vi "Write Objects.vi"(8 "error in (no error)":errorcluster, 10 "objects":cluster{"object ID":u8, "value":string}[](array[cluster]) {"object ID" format="%x"}, 11 "standard data model in":refnum<class "Standard Data Model.lvclass">) -> (0 "error out":errorcluster, 3 "standard data model out":refnum<class "Standard Data Model.lvclass">)   [LabVIEW 2017, in "SubVIs.lvlib" / "Standard Data Model.lvclass"]
doc: "Writes objects to the device model."
uses:
  <vilib>/Modbus/subvis/Data and Functions/Standard Data Model/Standard Data Model.lvclass
  <vilib>/Modbus/subvis/Data and Functions/Standard Data Model/Standard Data Model.lvclass/Standard Data Model.ctl
  <vilib>/Modbus/subvis/Data and Functions/Device Data Model/Device Data Model.lvclass
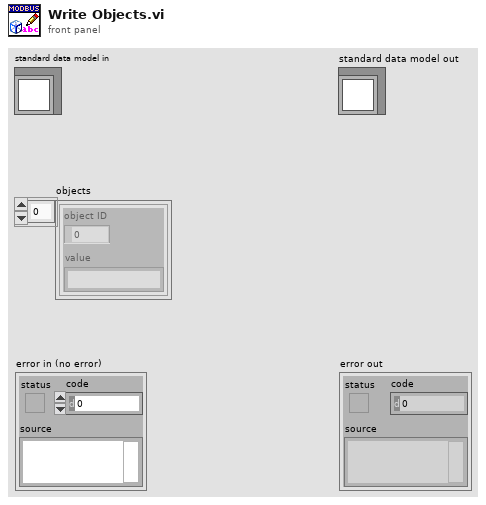
[diagram p1: front panel]
types:
  T1 = typedef "SubVIs.lvlib/Device Data Model.lvclass/Identification Parameters.ctl" = cluster{"object ID":u8, "value":string}
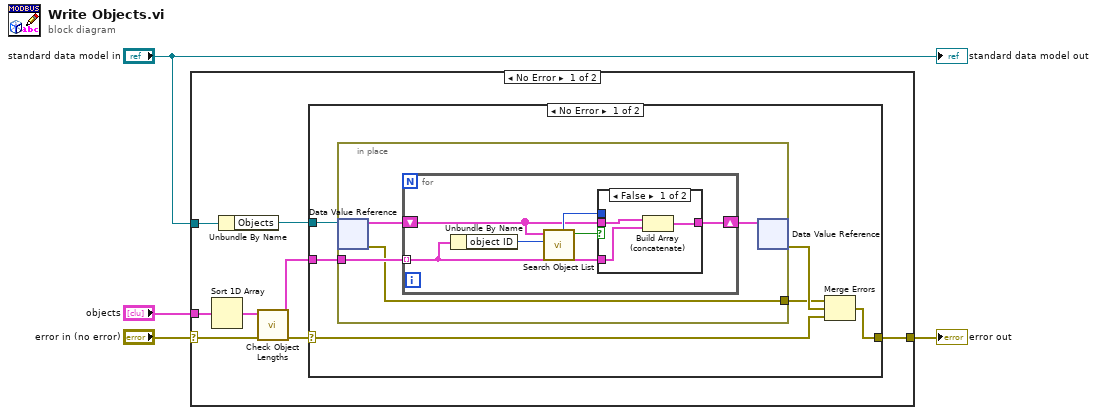
[diagram p0: block diagram]
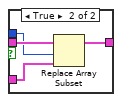
[diagram p2: hidden frame]
diagram:
  n1 = case shown="No Error" "error in (no error)" {
    selector: "error in (no error)" -> [w5 w37]
    tunnel: "objects" -> [w12 _]
    tunnel: "standard data model in" -> [w10 _]
    tunnel: [w7 w37] -> w2
    frame No Error {
      n2 = Sort 1D Array(array=w12) -> (sorted array=w9:cluster{"object ID":u8, "value":string}[])
      n3 = Unbundle By Name(w10) -> ("Objects"=w11:refnum<data-value>)
      n4 = call <vilib>:"Check Object Lengths.vi"("error in (no error)"=w5, "objects in"=w9) -> ("error out"=w8:errorcluster, "objects out"=w6:cluster{"object ID":u8, "value":string}[])  [unwired: 8 in]
      n5 = case shown="No Error" w8 {
        selector: w8 -> [w13 w36]
        tunnel: [w18 w36] -> w7
        tunnel: w11 -> [w17 _]
        tunnel: w6 -> [w16 _]
        frame No Error {
          n6 = in-place {
            in-place-border: w16 -> [w20]
            in-place-border: [w19] -> w14
            n7 = in-place-dvr #1(w17) -> (w22:T1[], w19:errorcluster)
            n8 = for {
              shift-right: [w24] -> w21
              shift-left: w22 -> [w25]
              tunnel: w20 -> [w23] mode=indexing
              n9 = Unbundle By Name(w23) -> ("object ID"=w28:u8)
              n10 = call <vilib>:"Search Object List.vi"("object ID"=w28, "objects"=w25) -> ("found?"=w27:bool, "index"=w26:i32)  [unwired: 7 in, 1 out]
              n11 = case shown="False" w27 {
                tunnel: w23 -> [w29 w32]
                tunnel: w26 -> [_ w33]
                tunnel: w25 -> [w31 w35]
                tunnel: [w30 w34] -> w24
                frame False {
                  n12 = Build Array (concatenate)(w31, w29) -> (w30:T1[])
                }
                frame True {
                  n13 = Replace Array Subset(array=w35, new element=w32, index=w33) -> (w34:T1[])
                }
              }
            }
            n14 = in-place-dvr #1(w21) -> (w15:errorcluster)  [unwired: 1 out]
          }
          n15 = Merge Errors(w14, w15, w13) -> (w18:errorcluster)
        }
        frame Error {
        }
      }
    }
    frame Error {
    }
  }
  "error out" <- w2
  "standard data model out" <- "standard data model in"
